vi "uView_fp.insert.vi"(8 "error in (no error)":errorcluster, 10 "subPanel":refnum<vi>, 11 "uView Transport":refnum<class "uTransport_uActor.lvclass">) -> (0 "error out":errorcluster)   [LabVIEW 2023, in "uFramework_pack_uActor.lvlib" / "uView.lvclass"]
doc: "insert the View into the provided subpanel."
uses:
  uView.lvclass
  Bin/uFramework.lvlibp/uTransport_uActor/uTransport_uActor.lvclass
  Bin/uData.lvlibp/uData.lvclass
  Bin/uFramework.lvlibp/uActor/uActor.lvclass
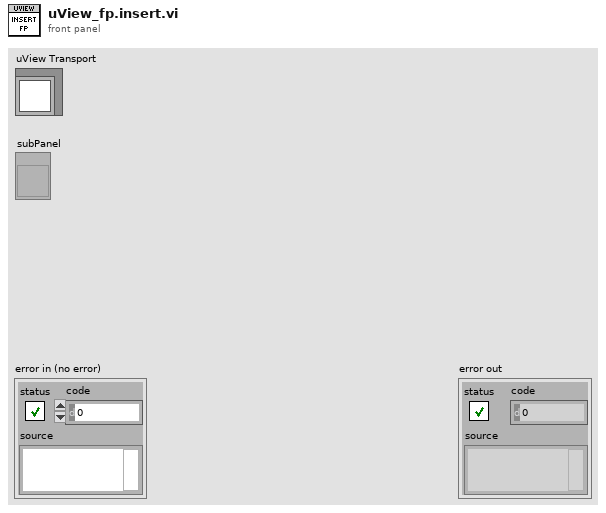
[diagram p1: front panel]
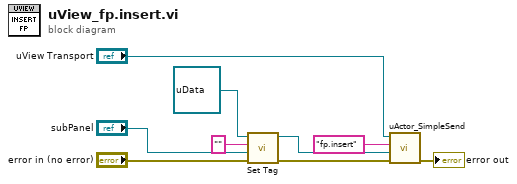
[diagram p0: block diagram]
diagram:
  n1 = call "Set Tag.vi"("error in (no error)"="error in (no error)", "Variant"="subPanel", "tag (case insensitive)"="", "uData in"=refnum<class "uData.lvclass"> refnum) -> ("error out"=w8:errorcluster, "uData out"=w4:refnum<class "uData.lvclass">)  [unwired: 5 in, 1 out]
  n2 = call "uActor_SimpleSend.vi"("error in (no error)"=w8, "Payload"=w4, "Msg"="fp.insert", "uActor Transport"="uView Transport") -> ("error out"=→"error out":errorcluster)  [unwired: 7 in]
